vi "Interferance_Test_New.vi"   [LabVIEW 2019]
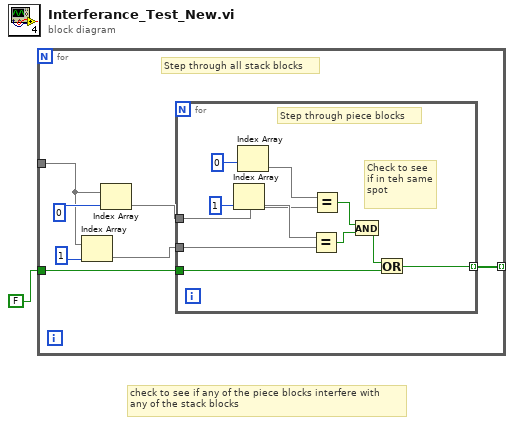
[diagram p0: block diagram]
diagram:
  # "check to see if any of the piece blocks interfere with \nany of the stack blocks"
  n1 = for {
    tunnel: _ -> [w5]
    tunnel: FALSE -> [w3]
    tunnel: [w2] -> _ mode=indexing
    # "Step through all stack blocks"
    n2 = Index Array(array=w5, index=1) -> (element=w6)
    n3 = Index Array(array=w5, index=0) -> (element=w4)
    n4 = for {
      tunnel: w6 -> [w15]
      tunnel: w4 -> [w14]
      tunnel: w3 -> [w10]
      tunnel: [w9] -> w2 mode=indexing
      # "Check to see if in teh same spot"
      # "Step through piece blocks"
      n5 = Index Array(index=1) -> (element=w16)  [unwired: 1 in]
      n6 = Index Array(index=0) -> (element=w13)  [unwired: 1 in]
      n7 = Equal?(x=w16, y=w15) -> (x = y?=w19:bool)
      n8 = Equal?(x=w13, y=w14) -> (x = y?=w17:bool)
      n9 = And(x=w17, y=w19) -> (x .and. y?=w18:bool)
      n10 = Or(x=w18, y=w10) -> (x .or. y?=w9:bool)
    }
  }
